vi "CONV String to 1D Fractional.vi"(0 "String":string, 1 "Delimiter (,)":string=",") -> (6 "1-D Fractional":dbl[](array[numeric]) format="%.2f")   [LabVIEW 2012]
doc: "This routine converts a string list to a 1-D DBL Precision Fractional array. String input may or may not have a trailing delimiter."
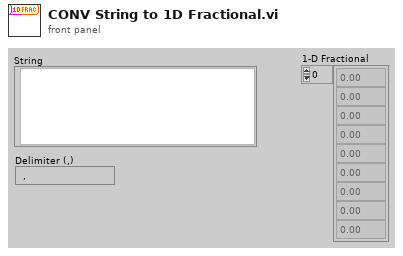
[diagram p1: front panel]
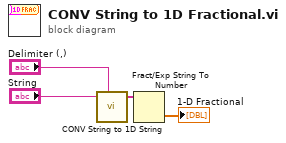
[diagram p0: block diagram]
diagram:
  n1 = call "CONV String to 1D String.vi"("String"="String", "Delimiter (,)"="Delimiter (,)") -> ("1-D String"=w1:string[])  [unwired: 7 out]
  n2 = Fract/Exp String To Number(string=w1) -> (number=→"1-D Fractional":dbl[])  [unwired: 1 in, 3 out]
